vi "MEM IO Read__ogtk.vi"   [LabVIEW 2018]
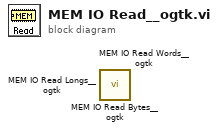
[diagram p0: block diagram]
diagram:
  n1 = call <userlib>:"MEM IO Read Bytes__ogtk.vi"() -> ()  [unwired: 6 in, 2 out]
  n2 = call <userlib>:"MEM IO Read Words__ogtk.vi"() -> ()  [unwired: 6 in, 2 out]
  n3 = call <userlib>:"MEM IO Read Longs__ogtk.vi"() -> ()  [unwired: 6 in, 2 out]
